vi "Extract Position Orientation.vi"(8 "Error In":errorcluster, 10 "Tracker":T1, 11 "Rigid Body Data":T3[](array[typedef])) -> (0 "Error Out":errorcluster, 3 "Rigid Body":T4)   [LabVIEW 2017]
uses:
  Controls/Rigid Body Info.ctl
  Controls/Position.ctl
  Controls/Orientation.ctl
  Controls/Raw Rigid Body Data.ctl
  <vilib>/Analysis/Matrix/Datatypes/RealMatrix.ctl
  Controls/Tracker Type.ctl
  <vilib>/Analysis/baseanly.llb/Real A x B.vi
  <vilib>/Analysis/_algsub.llb/Vector Norm.vi
  <vilib>/Analysis/_algsub.llb/Real Vector Norm.vi
  <vilib>/Analysis/baseanly.llb/Outer Product.vi
  <vilib>/Analysis/baseanly.llb/Real Outer Product.vi
  <vilib>/robotics/Kinematics/Create Lie Group Matrix.vi
  <vilib>/Analysis/Matrix/Numeric/Multiply/Multiply.vi
  <vilib>/Analysis/Matrix/Numeric/Multiply/Multiply - RM,R.vi
  <vilib>/Analysis/Matrix/Numeric/Multiply/Multiply - R,RM.vi
  <vilib>/Analysis/Matrix/Numeric/Add/Add.vi
  <vilib>/Analysis/Matrix/Numeric/Add/Add - RM,RM.vi
  <vilib>/Analysis/baseanly.llb/Real Inverse Matrix.vi
  <vilib>/robotics/Kinematics/Rotation Matrix to Angle Vector.vi
  <vilib>/robotics/Kinematics/NI_Kinematics.lvlib
  <vilib>/Analysis/NI_AALBase.lvlib
  <vilib>/Analysis/Matrix/NI_Matrix.lvlib
panel:
  out "world_T^patient":T2
  out "world_T^probe":T2
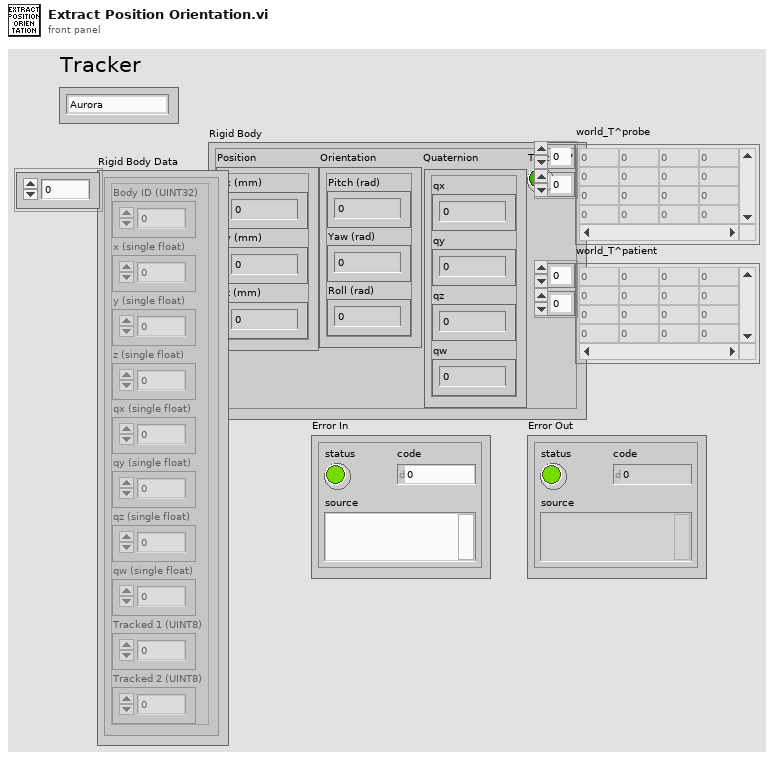
[diagram p1: front panel]
types:
  T1 = typedef "Tracker Type.ctl" = enum16{"Aurora", "OptiTrack"}
  T2 = typedef "NI_Matrix.lvlib/RealMatrix.ctl" = dbl[][]
  T3 = typedef "Raw Rigid Body Data.ctl" = cluster{"Body ID (UINT32)":u32, "x (single float)":sgl, "y (single float)":sgl, "z (single float)":sgl, "qx (single float)":sgl, "qy (single float)":sgl, "qz (single float)":sgl, "qw (single float)":sgl, "Tracked 1 (UINT8)":u8, "Tracked 2 (UINT8)":u8}
  T4 = typedef "Rigid Body Info.ctl" = cluster{"Position":T5, "Orientation":T6, "Quaternion":cluster{"qx":sgl, "qy":sgl, "qz":sgl, "qw":sgl}, "Tracked?":bool}
  T5 = typedef "Position.ctl" = cluster{"x (mm)":sgl, "y (mm)":sgl, "z (mm)":sgl}
  T6 = typedef "Orientation.ctl" = cluster{"Pitch (rad)":sgl, "Yaw (rad)":sgl, "Roll (rad)":sgl}
  T7 = typedef "NI_Kinematics.lvlib/Quaternion.ctl" = dbl[]
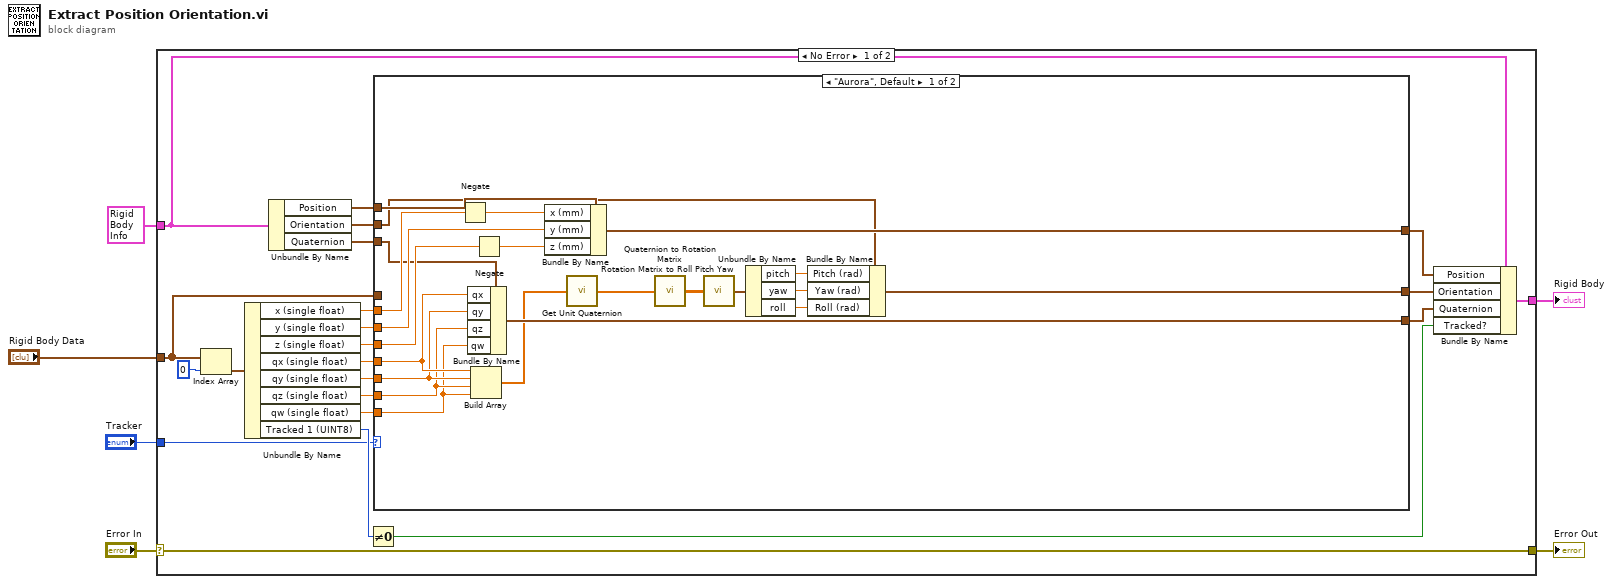
[diagram p0: block diagram]
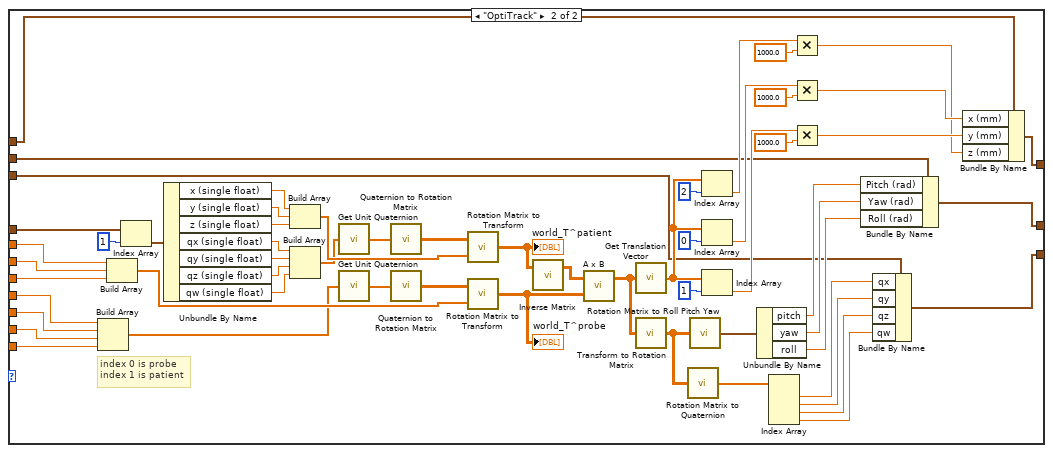
[diagram p2: hidden frame]
diagram:
  n1 = case shown="No Error" "Error In" {
    selector: "Error In" -> [w19 w109]
    tunnel: [w28 w110] -> w6
    tunnel: T4 {"Position"={"x (mm)"=0.0, "y (mm)"=0.0, "z (mm)"=0.0}, "Orientation"={"Pitch (rad)"=-180.0, "Yaw (rad)"=-0.0, "Roll (rad)"=-180.0}, "Quaternion"={"qx"=0.0, "qy"=0.0, "qz"=0.0, "qw"=0.0}, "Tracked?"=FALSE} ("Rigid Body") -> [w26 w110]
    tunnel: "Rigid Body Data" -> [w14 _]
    tunnel: [w19 w109] -> w2
    tunnel: "Tracker" -> [w7 _]
    frame No Error {
      n2 = Index Array(array=w14, index=0) -> (element=w20:T3)
      n3 = Unbundle By Name(w20) -> ("x (single float)"=w18:sgl, "y (single float)"=w17:sgl, "z (single float)"=w16:sgl, "qx (single float)"=w22:sgl, "qy (single float)"=w23:sgl, "qz (single float)"=w24:sgl, "qw (single float)"=w25:sgl, "Tracked 1 (UINT8)"=w21:u8)
      n4 = Unbundle By Name(w26) -> ("Position"=w11:T5, "Orientation"=w13:T6, "Quaternion"=w9:cluster{"qx":sgl, "qy":sgl, "qz":sgl, "qw":sgl})
      n5 = Not Equal To 0?(x=w21) -> (x != 0?=w27:bool)
      n6 = case shown="\"Aurora\", Default" w7 {
        tunnel: w25 -> [w33 w104]
        tunnel: w24 -> [w34 w103]
        tunnel: w23 -> [w35 w102]
        tunnel: w22 -> [w41 w101]
        tunnel: w18 -> [w49 w100]
        tunnel: w17 -> [w48 w99]
        tunnel: w16 -> [w47 w98]
        tunnel: w14 -> [_ w93]
        tunnel: w13 -> [w45 w71]
        tunnel: [w39 w67] -> w12
        tunnel: w11 -> [w50 w66]
        tunnel: [w46 w62] -> w10
        tunnel: w9 -> [w44 w61]
        tunnel: [w40 w56] -> w8
        frame "Aurora", Default {
          n7 = Negate(x=w49) -> (-x=w29:sgl)
          n8 = Bundle By Name(cluster=w44, "qx"=w41, "qy"=w35, "qz"=w34, "qw"=w33) -> (w40:cluster{"qx":sgl, "qy":sgl, "qz":sgl, "qw":sgl})
          n9 = Build Array(w41, w35, w34, w33) -> (w31:sgl[])
          n10 = Negate(x=w47) -> (-x=w32:sgl)
          n11 = Bundle By Name(cluster=w50, "x (mm)"=w29, "y (mm)"=w48, "z (mm)"=w32) -> (w46:T5)
          n12 = call <vilib>:"Get Unit Quaternion.vi"("quaternion"=w31) -> ("unit quaternion"=w30:T7)
          n13 = call <vilib>:"Quaternion to Rotation Matrix.vi"("quaternion"=w30) -> ("rotation matrix"=w42:T2)
          n14 = call <vilib>:"Rotation Matrix to Roll Pitch Yaw.vi"("rotation matrix"=w42) -> ("angles"=w43:cluster{"roll":dbl, "pitch":dbl, "yaw":dbl})
          n15 = Unbundle By Name(w43) -> ("pitch"=w36:dbl, "yaw"=w37:dbl, "roll"=w38:dbl)
          n16 = Bundle By Name(cluster=w45, "Pitch (rad)"=w36, "Yaw (rad)"=w37, "Roll (rad)"=w38) -> (w39:T6)
        }
        frame "OptiTrack" {
          # "index 0 is probe\nindex 1 is patient"
          n17 = Build Array(w101, w102, w103, w104) -> (w52:sgl[])
          n18 = Build Array(w100, w99, w98) -> (w96:sgl[])
          n19 = Index Array(array=w93, index=1) -> (element=w94:T3)
          n20 = Unbundle By Name(w94) -> ("x (single float)"=w92:sgl, "y (single float)"=w91:sgl, "z (single float)"=w90:sgl, "qx (single float)"=w89:sgl, "qy (single float)"=w88:sgl, "qz (single float)"=w86:sgl, "qw (single float)"=w87:sgl)
          n21 = Build Array(w92, w91, w90) -> (w85:sgl[])
          n22 = Build Array(w89, w88, w86, w87) -> (w54:sgl[])
          n23 = call <vilib>:"Get Unit Quaternion.vi"("quaternion"=w54) -> ("unit quaternion"=w53:T7)
          n24 = call <vilib>:"Get Unit Quaternion.vi"("quaternion"=w52) -> ("unit quaternion"=w51:T7)
          n25 = call <vilib>:"Quaternion to Rotation Matrix.vi"("quaternion"=w53) -> ("rotation matrix"=w55:T2)
          n26 = call <vilib>:"Quaternion to Rotation Matrix.vi"("quaternion"=w51) -> ("rotation matrix"=w97:T2)
          n27 = call <vilib>:"Rotation Matrix to Transform.vi"("translation vector"=w85, "rotation matrix"=w55) -> ("transform"=w80:T2)
          "world_T^patient" <- w80
          n28 = call <vilib>:"Rotation Matrix to Transform.vi"("translation vector"=w96, "rotation matrix"=w97) -> ("transform"=w79:T2)
          "world_T^probe" <- w79
          n29 = call-poly <vilib>:"Inverse Matrix.vi"("Input Matrix"=w80) -> ("Inverse Matrix"=w74:T2)  [unwired: 1 in, 1 out]
          n30 = call-poly <vilib>:"A x B.vi"("B"=w79, "A"=w74) -> ("A x B"=w78:T2)  [unwired: 1 out]
          n31 = call <vilib>:"Get Translation Vector.vi"("transform"=w78) -> ("translation vector"=w84:dbl[])
          n32 = call <vilib>:"Transform to Rotation Matrix.vi"("transform"=w78) -> ("rotation matrix"=w73:T2)
          n33 = call <vilib>:"Rotation Matrix to Quaternion.vi"("rotation matrix"=w73) -> ("quaternion"=w72:T7)
          n34 = call <vilib>:"Rotation Matrix to Roll Pitch Yaw.vi"("rotation matrix"=w73) -> ("angles"=w105:cluster{"roll":dbl, "pitch":dbl, "yaw":dbl})
          n35 = Index Array(array=w84, index=2) -> (element=w75:dbl)
          n36 = Index Array(array=w84, index=0) -> (element=w76:dbl)
          n37 = Index Array(array=w84, index=1) -> (element=w77:dbl)
          n38 = Unbundle By Name(w105) -> ("pitch"=w70:dbl, "yaw"=w69:dbl, "roll"=w68:dbl)
          n39 = Index Array(array=w72) -> (element #1=w60:dbl, element #2=w59:dbl, element #3=w58:dbl, element #4=w57:dbl)  [unwired: 4 in]
          n40 = Multiply(x=w75, y=sgl 1000.0) -> (x*y=w63:dbl)
          n41 = Multiply(x=w76, y=sgl 1000.0) -> (x*y=w65:dbl)
          n42 = Multiply(x=w77, y=sgl 1000.0) -> (x*y=w64:dbl)
          n43 = Bundle By Name(cluster=w71, "Pitch (rad)"=w70, "Yaw (rad)"=w69, "Roll (rad)"=w68) -> (w67:T6)
          n44 = Bundle By Name(cluster=w61, "qx"=w60, "qy"=w59, "qz"=w58, "qw"=w57) -> (w56:cluster{"qx":sgl, "qy":sgl, "qz":sgl, "qw":sgl})
          n45 = Bundle By Name(cluster=w66, "x (mm)"=w65, "y (mm)"=w64, "z (mm)"=w63) -> (w62:T5)
        }
      }
      n46 = Bundle By Name(cluster=w26, "Position"=w10, "Orientation"=w12, "Quaternion"=w8, "Tracked?"=w27) -> (w28:T4)
    }
    frame Error {
    }
  }
  "Rigid Body" <- w6
  "Error Out" <- w2
